vi "Cycle Average and RMS N chan.vi"(6 "percent level settings":T3={"method"=enum."auto select", "histogram size"=256, "histogram method"=enum."mode", "reserved"=1.0} {"reserved" format="%0.2f"}, 7 "cycle number (1)":i32=1 min=1, 8 "error in (no error)":errorcluster, 9 "reference levels":T2={"high ref level"=90.0, "mid ref level"=50.0, "low ref level"=10.0, "ref units"=1} {"ref units" items=["absolute", "percent"]; "high ref level" format="%.2p"; "low ref level" format="%.2p"; "mid ref level" format="%.2p"}, 11 "signal(s) in":waveform(dbl)[](array[waveform])) -> (0 "error out":errorcluster, 2 "cycle RMS":dbl[](array[numeric]) format="%.2p", 3 "cycle average":dbl[](array[numeric]) format="%.2p", 4 "measurement info":T1(array[cluster]))   [LabVIEW 2020, in "NI_MAPro.lvlib"]
doc: "Returns the average and RMS levels of a selected cycle of a periodic waveform or an array of periodic waveforms. Wire data to the <B>signal in</B> input to determine the polymorphic instance to use or manually select the instance."
uses:
  NI_MAPro.lvlib
  NI_MABase.lvlib
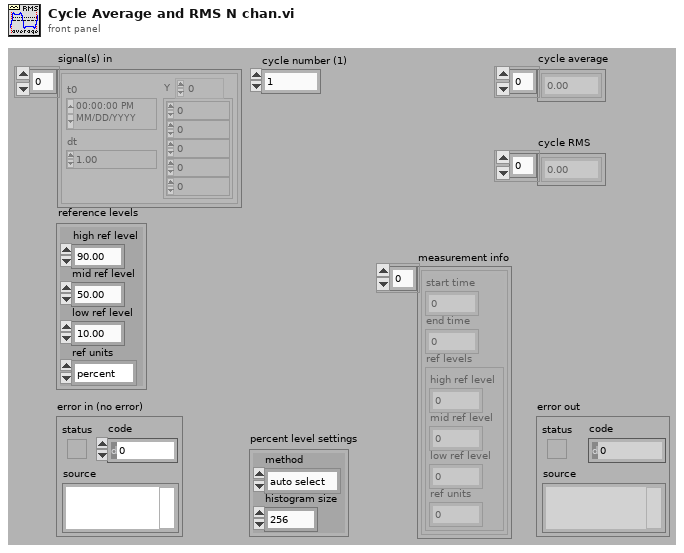
[diagram p1: front panel]
types:
  T1 = cluster{"start time":dbl, "end time":dbl, "ref levels":cluster{"high ref level":dbl, "mid ref level":dbl, "low ref level":dbl, "ref units":u16}}[]
  T2 = cluster{"high ref level":dbl, "mid ref level":dbl, "low ref level":dbl, "ref units":u16}
  T3 = cluster{"method":enum32{"histogram", "peak", "auto select"}, "histogram size":i32, "histogram method":enum16{"mode"}, "reserved":dbl}
  T4 = cluster{"start time":dbl, "end time":dbl, "ref levels":cluster{"high ref level":dbl, "mid ref level":dbl, "low ref level":dbl, "ref units":u16}}
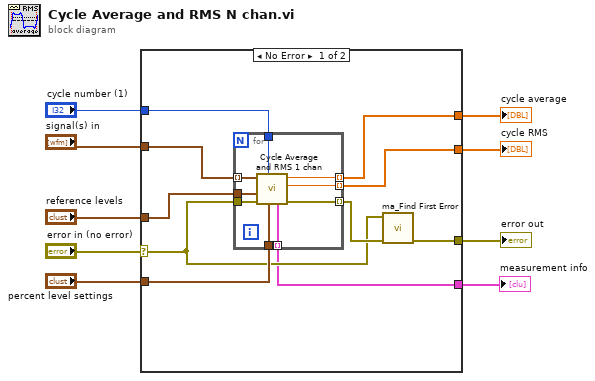
[diagram p0: block diagram]
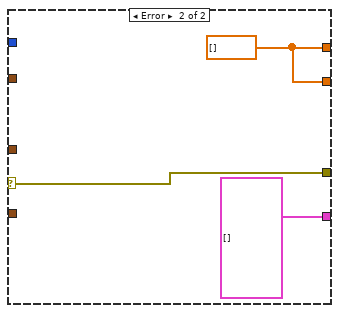
[diagram p2: hidden frame]
diagram:
  n1 = case shown="No Error" "error in (no error)" {
    selector: "error in (no error)" -> [w14 w31]
    tunnel: "percent level settings" -> [w18 _]
    tunnel: [w13 w31] -> w7
    tunnel: "signal(s) in" -> [w19 _]
    tunnel: [w17 w30] -> w5
    tunnel: [w16 w30] -> w4
    tunnel: "reference levels" -> [w12 _]
    tunnel: "cycle number (1)" -> [w11 _]
    tunnel: [w10 T1 []] -> w1
    frame No Error {
      n2 = for {
        tunnel: w14 -> [w28]
        tunnel: w18 -> [w27]
        tunnel: [w26] -> w15 mode=indexing
        tunnel: [w25] -> w17 mode=indexing
        tunnel: [w24] -> w16 mode=indexing
        tunnel: w19 -> [w23] mode=indexing
        tunnel: w12 -> [w22]
        tunnel: w11 -> [w21]
        tunnel: [w20] -> w10 mode=indexing
        n3 = call "Cycle Average and RMS 1 chan.vi"("percent level settings"=w27, "cycle number (1)"=w21, "error in (no error)"=w28, "reference levels"=w22, "signal in"=w23) -> ("error out"=w26:errorcluster, "cycle RMS"=w24:dbl, "cycle average"=w25:dbl, "measurement info"=w20:T4)  [unwired: 1 in, 2 out]
      }
      n4 = call "ma_Find First Error.vi"("error array in"=w15, "error in 1 (no error)"=w14) -> ("error out"=w13:errorcluster)  [unwired: 2 in, 3 out]
    }
    frame Error {
      w30 = dbl[] []
    }
  }
  "error out" <- w7
  "cycle average" <- w5
  "cycle RMS" <- w4
  "measurement info" <- w1
